vi "Find peaks.vi"(8 "Error In":errorcluster, 9 "Channel names":string[](array[string])=["X", "Y", "Frequency"], 10 "group name":string, 11 "tdms file":refnum<k34>) -> (0 "Error Out":errorcluster, 1 "Width":dbl[](array[numeric]) format="%#_6p", 2 "Peak F":dbl[](array[numeric]) format="%#_8p", 3 "tdms file out":refnum<k34>, 4 "Peak Amplitude":dbl[](array[numeric]))   [LabVIEW 2015]
uses:
  <vilib>/Analysis/3filter.llb/Filter Passband Type.ctl
  <vilib>/Analysis/3filter.llb/Butterworth Filter (CDB).vi
  <vilib>/Analysis/NI_AAL_SigProc.lvlib
  <vilib>/Analysis/NI_AALBase.lvlib
panel:
  in  "cutoff freq: fl":dbl=0.12500000000000006 format="%.4p"
  out "2nd Derivatives":dbl[](array[numeric])
  out "Locations":dbl[](array[numeric])
  in  "width":dbl=150.0 format="%#_6p"
  in  "threshold":dbl=0.15 format="%0.2f"
  out "XY Graph":cluster{dbl[], dbl[]}[](graph)
  # "of max"
  # "Hz"
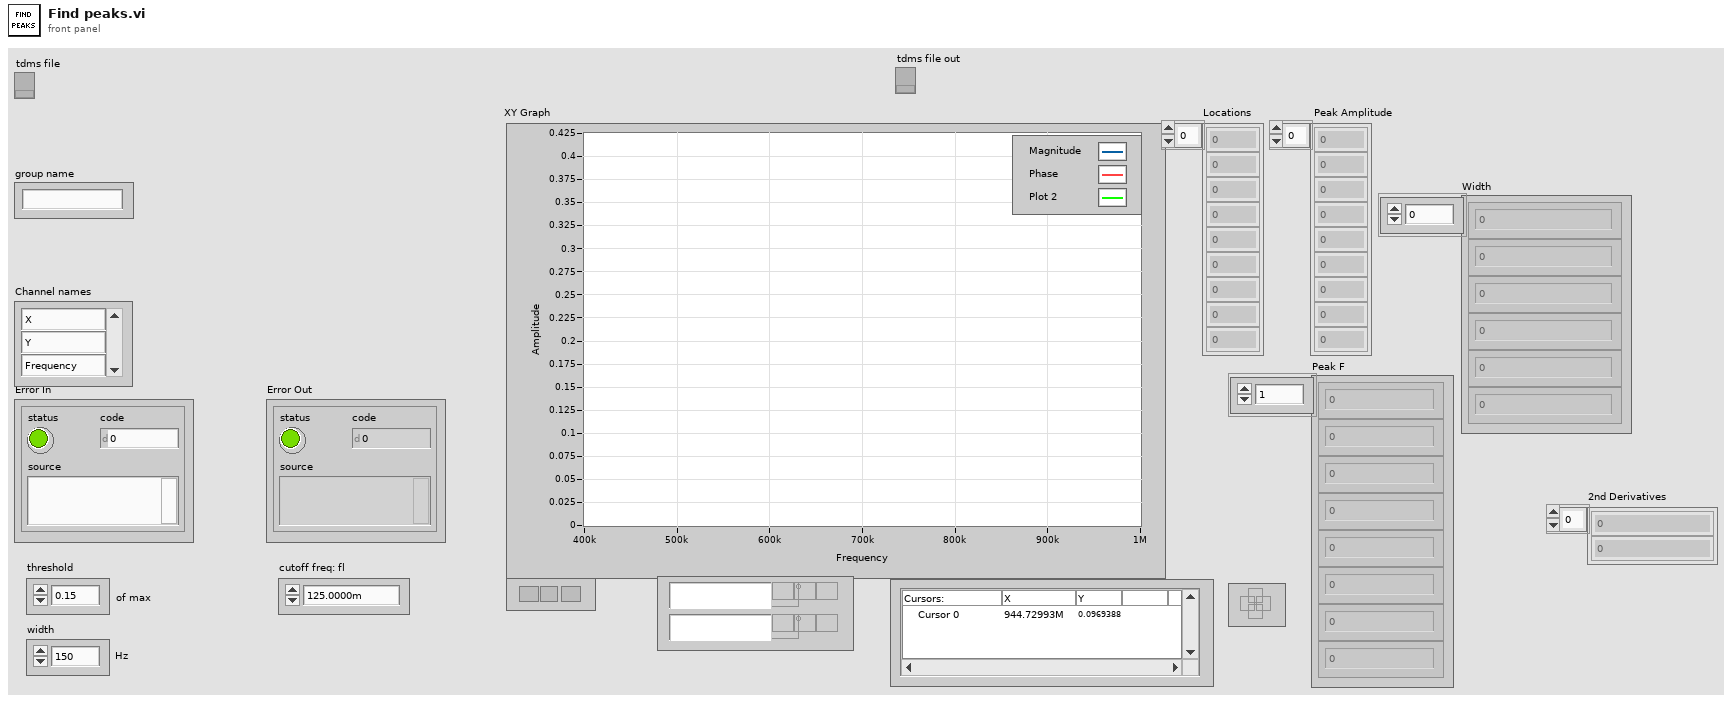
[diagram p1: front panel]
types:
  T1 = typedef "NI_AALBase.lvlib/Filter Passband Type.ctl" = enum32{"Lowpass", "Highpass", "Bandpass", "Bandstop"}
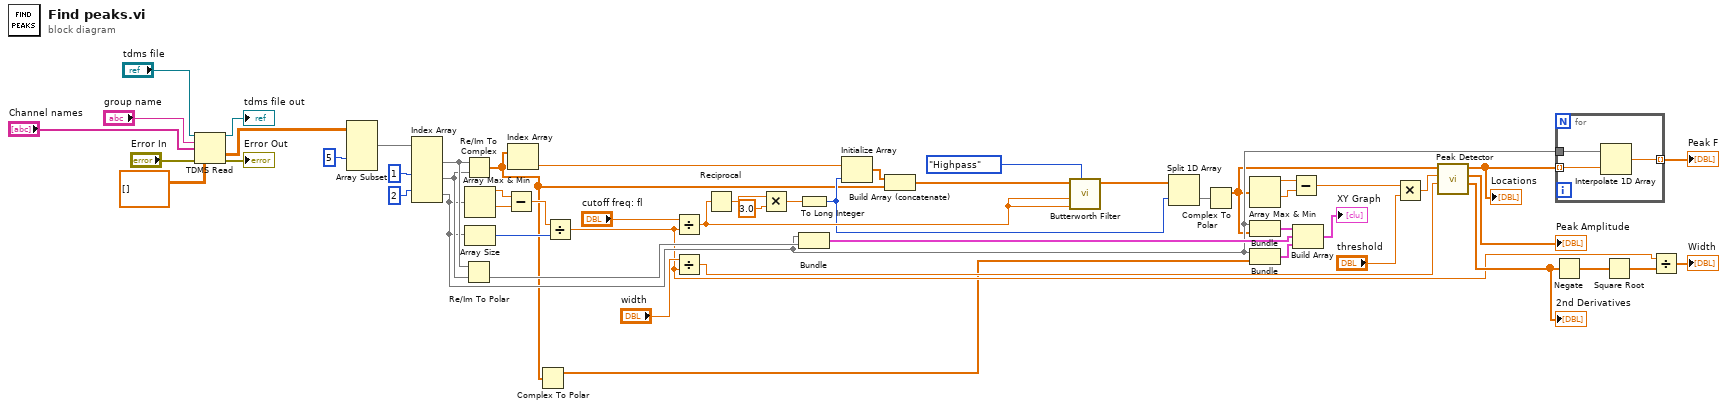
[diagram p0: block diagram]
diagram:
  n1 = TDMS Read(0:"tdms file", 5:"group name", 7:"Channel names", 11:"Error In", 12:dbl[][] []) -> (4:→"tdms file out":refnum<k34>, 10:w6:dbl[][], 15:→"Error Out":errorcluster)  [unwired: 3 in, 3 out]
  n2 = Array Subset(array=w6, index (col)=5 ("index")) -> (w5:dbl[][])  [unwired: 3 in]
  n3 = Index Array(array=w5, index (row) #2=1 ("index (row)"), index (row) #3=2 ("index (row)")) -> (element #1=w22:dbl[], element #2=w21:dbl[], element #3=w20:dbl[])  [unwired: 4 in]
  n4 = Re/Im To Complex(1:w21, 2:w22) -> (0:w2:cdb[])
  n5 = Re/Im To Polar(2:w21, 3:w22) -> (0:w45:dbl[])  [unwired: 1 out]
  n6 = Array Max & Min(array=w20) -> (max value=w44:dbl, min value=w43:dbl)  [unwired: 2 out]
  n7 = Array Size(array=w20) -> (size(s)=w42:i32)
  n8 = Subtract(x=w44, y=w43) -> (x-y=w31:dbl)
  n9 = Index Array(array=w2) -> (element=w15:cdb)  [unwired: 1 in]
  n10 = Complex To Polar(r * e^(i*theta)=w2) -> (r=w1:dbl[])  [unwired: 1 out]
  n11 = Divide(x=w31, y=w42) -> (x/y=w16:dbl)
  n12 = Divide(x="cutoff freq: fl", y=w16) -> (x/y=w14:dbl)
  n13 = Divide(x="width", y=w16) -> (x/y=w19:dbl)
  n14 = Reciprocal(x=w14) -> (1/x=w13:dbl)
  n15 = Multiply(x=w13, y=3.0) -> (x*y=w11:dbl)
  n16 = To Long Integer(number=w11) -> (32bit integer=w9:i32)
  n17 = Bundle(w20, w45) -> (w47:cluster{dbl[], dbl[]})  [unwired: 1 in]
  n18 = Initialize Array(w15, w9) -> (w7:cdb[])
  n19 = Build Array (concatenate)(w7, w2) -> (w10:cdb[])
  n20 = call-poly <vilib>:"Butterworth Filter.vi"("filter type"=Filter_Passband_Type."Highpass", "low cutoff freq: fl"=w14, "high cutoff freq: fh"=w14, "X"=w10) -> ("Filtered X"=w23:cdb[])  [unwired: 4 in, 1 out]
  n21 = Split 1D Array(array=w23, index=w9) -> (second subarray=w8:cdb[])  [unwired: 1 out]
  n22 = Complex To Polar(r * e^(i*theta)=w8) -> (r=w3:dbl[])  [unwired: 1 out]
  n23 = Array Max & Min(array=w3) -> (max value=w40:dbl, min value=w39:dbl)  [unwired: 2 out]
  n24 = Bundle(w20, w3) -> (w48:cluster{dbl[], dbl[]})  [unwired: 1 in]
  n25 = Bundle(w20, w1) -> (w17:cluster{dbl[], dbl[]})  [unwired: 1 in]
  n26 = Subtract(x=w40, y=w39) -> (x-y=w38:dbl)
  n27 = Build Array(w48, w47, w17) -> (→"XY Graph":cluster{dbl[], dbl[]}[])
  n28 = Multiply(x=w38, y="threshold") -> (x*y=w36:dbl)
  n29 = call <vilib>:"Peak Detector.vi"("width"=w19, "threshold"=w36, "X"=w3) -> ("2nd Derivatives"=w32:dbl[], "Amplitudes"=→"Peak Amplitude":dbl[], "Locations"=w34:dbl[])  [unwired: 4 in, 2 out]
  "Locations" <- w34
  "2nd Derivatives" <- w32
  n30 = Negate(x=w32) -> (-x=w29:dbl[])
  n31 = for {
    tunnel: w34 -> [w56] mode=indexing
    tunnel: w20 -> [w57]
    tunnel: [w55] -> w33 mode=indexing
    n32 = Interpolate 1D Array(1:w56, 2:w57) -> (0:w55:dbl)
  }
  "Peak F" <- w33
  n33 = Square Root(x=w29) -> (sqrt(x)=w28:dbl[])
  n34 = Divide(x=w16, y=w28) -> (x/y=→"Width":dbl[])
